vi "read_y.vi"(8 "error in (no error)":errorcluster, 11 "GaussianProcessRegressor in":refnum<class "GaussianProcessRegressor.lvclass">) -> (0 "error out":errorcluster, 2 "y":dbl[](array[numeric]), 3 "GaussianProcessRegressor out":refnum<class "GaussianProcessRegressor.lvclass">)   [LabVIEW 2020, in "GaussianProcessRegressor.lvclass"]
uses:
  GaussianProcessRegressor.lvclass
  GaussianProcessRegressor.lvclass/GaussianProcessRegressor.ctl
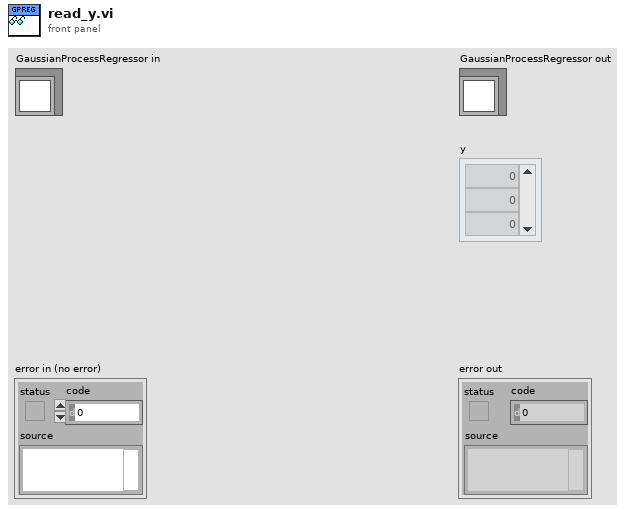
[diagram p1: front panel]
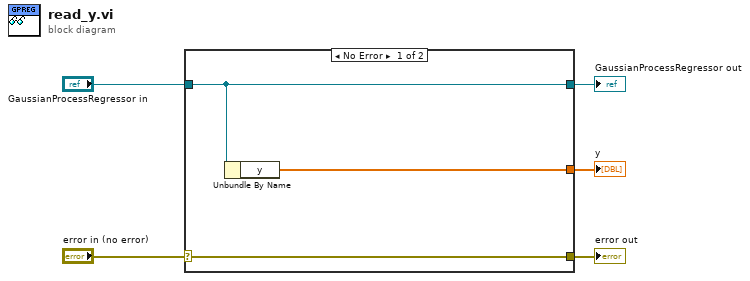
[diagram p0: block diagram]
diagram:
  n1 = case shown="No Error" "error in (no error)" {
    selector: "error in (no error)" -> [w8 w9]
    tunnel: [w8 w9] -> w4
    tunnel: [w7 w10] -> w2
    tunnel: "GaussianProcessRegressor in" -> [w7 w10]
    tunnel: [w6 _] -> w1
    frame No Error {
      n2 = Unbundle By Name(w7) -> ("y"=w6:dbl[])
    }
    frame Error {
    }
  }
  "error out" <- w4
  "GaussianProcessRegressor out" <- w2
  "y" <- w1
